vi "Initialize.vi"(7 "ChannelName":string="Setpoint.ch%d.SP", 8 "error in":errorcluster, 9 "Number of Channels":u32=1, 10 "Instance Name":string, 11 "OnOff Channels in":refnum<class "OnOff Channels.lvclass">) -> (0 "error out":errorcluster, 2 "Channel":T1[](array[typedef]), 3 "OnOff Channels out":refnum<class "OnOff Channels.lvclass">)   [LabVIEW 2023, in "OnOff Channels.lvclass"]
uses:
  OnOff Channels.lvclass
  <vilib>/ADAS Replay HIL/Channels/Tag Wrapper/Tag Wrapper.lvlib
  Utilities/Utilities.lvlib
  <vilib>/ADAS Replay HIL/Channels/Tag Wrapper/Polymorphic/Open Producer Tag (I32).vi
  <vilib>/ADAS Replay HIL/Channels/Tag Wrapper/Polymorphic/Set Default Value (Boolean).vi
  <vilib>/ADAS Replay HIL/Channels/Tag Wrapper/Polymorphic/Open Consumer Tag (Boolean).vi
  <vilib>/ADAS Replay HIL/Channels/Tag Wrapper/Polymorphic/Set Default Value (I32).vi
  Utilities/Channel.ctl
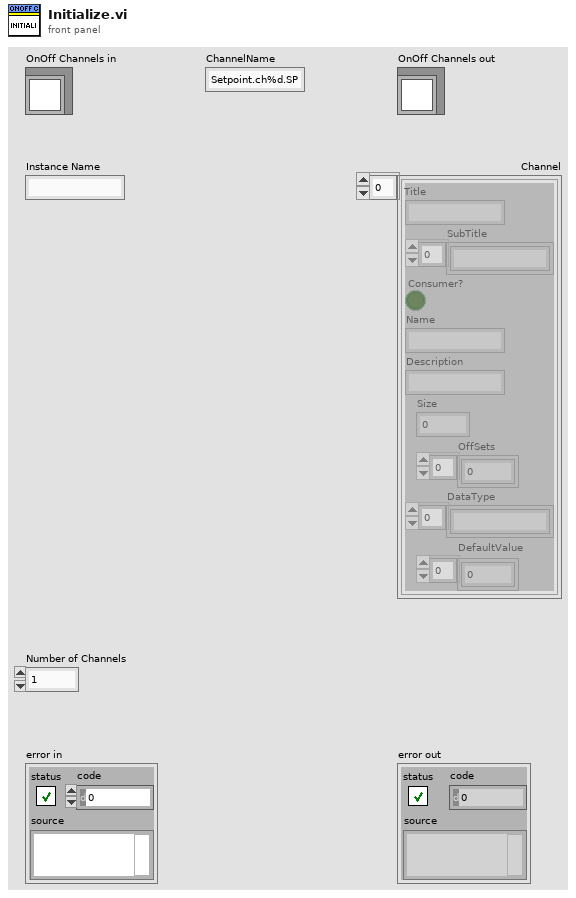
[diagram p1: front panel]
types:
  T1 = typedef "Utilities.lvlib/Channel.ctl" = cluster{"Title":string, "SubTitle":string[], "Consumer?":bool, "Name":string, "Description":string, "Size":i32, "OffSets":i32[], "DataType":string[], "DefaultValue":dbl[]}
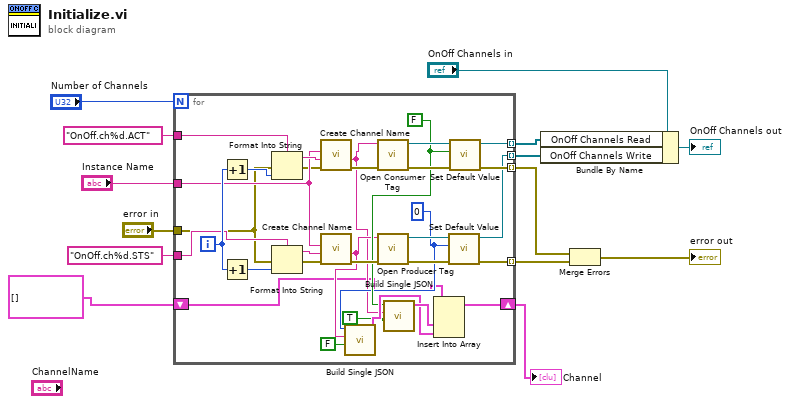
[diagram p0: block diagram]
diagram:
  n1 = for {
    N: "Number of Channels" -> [_]
    tunnel: "OnOff.ch%d.ACT" ("ChannelName") -> [w44]
    tunnel: "Instance Name" -> [w32]
    tunnel: "error in" -> [w25]
    tunnel: [w40] -> w12 mode=indexing
    tunnel: [w36] -> w13 mode=indexing
    tunnel: "OnOff.ch%d.STS" ("ChannelName") -> [w33]
    tunnel: [w30] -> w4 mode=indexing
    tunnel: [w29] -> w3 mode=indexing
    shift-right: [w22] -> w2
    shift-left: T1[] [] ("Channel") -> [w15]
    i -> [w34]
    w20 = 0 ("Default Value")
    w21 = FALSE ("Default Value")
    n2 = Increment(x=w34) -> (x+1=w45:i32)
    n3 = Increment(x=w34) -> (x+1=w35:i32)
    n4 = Format Into String(format string=w44, error in=w25, w45) -> (resulting string=w43:string, error out=w27:errorcluster)  [unwired: 1 in]
    n5 = Format Into String(format string=w33, error in=w25, w35) -> (resulting string=w31:string, error out=w26:errorcluster)  [unwired: 1 in]
    n6 = call "Create Channel Name.vi"("error in"=w27, "Channel Name"=w43, "Plugin Name"=w32) -> ("error out"=w28:errorcluster, "Data Channel Name"=w18:string)  [unwired: 7 in]
    n7 = call "Create Channel Name.vi"("error in"=w26, "Channel Name"=w31, "Plugin Name"=w32) -> ("error out"=w38:errorcluster, "Data Channel Name"=w19:string)  [unwired: 7 in]
    n8 = call "Build Single JSON.vi"("Consumer?"=FALSE, "ChannelName"=w19, "Single"=w20) -> ("Channel"=w23:T1)  [unwired: 7 in, 1 out]
    n9 = call-poly <vilib>:"Open Consumer Tag.vi"("error in"=w28, "Channel Name"=w18) -> ("error out"=w41:errorcluster, "ADAS HIL Channel"=w42:refnum<k21>)  [unwired: 8 in]
    n10 = call-poly <vilib>:"Open Producer Tag.vi"("error in"=w38, "Channel Name"=w19) -> ("error out"=w37:errorcluster, "ADAS HIL Channel"=w39:refnum<k21>)  [unwired: 8 in]
    n11 = call "Build Single JSON.vi"("Consumer?"=TRUE, "ChannelName"=w18, "Single"=w21) -> ("Channel"=w24:T1)  [unwired: 7 in, 1 out]
    n12 = Insert Into Array(array=w15, new element #1=w24, new element #2=w23) -> (w22:T1[])  [unwired: 1 in]
    n13 = call-poly <vilib>:"Set Default Value.vi"("error in"=w37, "Default Value"=w20, "ADAS HIL Channel in"=w39) -> ("error out"=w36:errorcluster, "ADAS HIL Channel out"=w29:refnum<k21>)  [unwired: 7 in]
    n14 = call-poly <vilib>:"Set Default Value.vi"("error in"=w41, "Default Value"=w21, "ADAS HIL Channel in"=w42) -> ("error out"=w40:errorcluster, "ADAS HIL Channel out"=w30:refnum<k21>)  [unwired: 7 in]
  }
  "Channel" <- w2
  n15 = Bundle By Name(cluster="OnOff Channels in", "OnOff Channels Read"=w4, "OnOff Channels Write"=w3) -> (→"OnOff Channels out":refnum<class "OnOff Channels.lvclass">)
  n16 = Merge Errors(w12, w13) -> (→"error out":errorcluster)
